vi "Local Vars.vi"() -> ()   [LabVIEW 2011]
panel:
  out "a+b+c+d":dbl
  out "loop count 2":i32
  out "x+y":dbl
  out "Loop count 1":i32
  in  "stop":bool
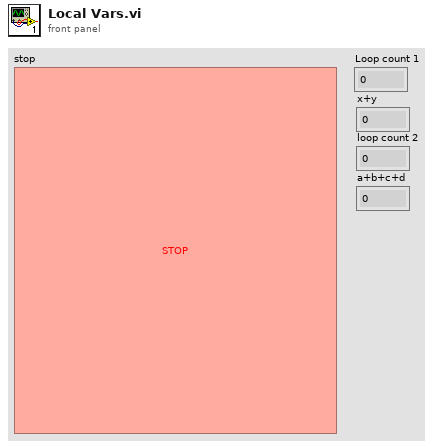
[diagram p1: front panel]
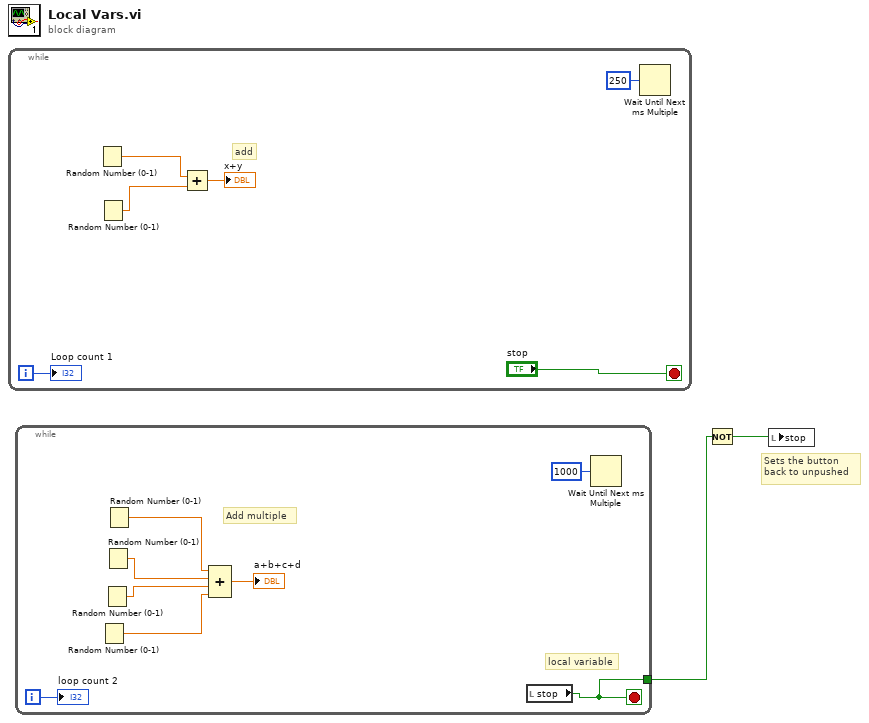
[diagram p0: block diagram]
diagram:
  # "Sets the button\nback to unpushed"
  n1 = while {
    i -> [w7]
    stop <- "stop" stop-if-true
    # "add"
    n2 = Random Number (0-1)() -> (number: 0 to 1=w6:dbl)
    n3 = Random Number (0-1)() -> (number: 0 to 1=w5:dbl)
    n4 = Add(x=w6, y=w5) -> (x+y=→"x+y":dbl)
    n5 = Wait Until Next ms Multiple(millisecond multiple=u32 250) -> ()  [unwired: 1 out]
    "Loop count 1" <- w7
  }
  n6 = while {
    tunnel: [w9] -> w1
    i -> [w15]
    stop <- w9 stop-if-true
    # "local variable"
    # "Add multiple"
    n7 = Random Number (0-1)() -> (number: 0 to 1=w11:dbl)
    n8 = Random Number (0-1)() -> (number: 0 to 1=w12:dbl)
    n9 = Random Number (0-1)() -> (number: 0 to 1=w13:dbl)
    n10 = Random Number (0-1)() -> (number: 0 to 1=w14:dbl)
    n11 = Compound Arithmetic op=ADD(w14, w13, w12, w11) -> (→"a+b+c+d":dbl)
    n12 = local read "stop"() -> (w9:bool)
    n13 = Wait Until Next ms Multiple(millisecond multiple=u32 1000) -> ()  [unwired: 1 out]
    "loop count 2" <- w15
  }
  n14 = Not(x=w1) -> (.not. x?=w2:bool)
  n15 = local write "stop"(w2) -> ()
